vi "SRV_Build Calculated Sensors Commands.vi"(8 "error in (no error)":errorcluster, 10 "Calculated Sensors Config":T2[](array[typedef]) {"Register" format="%.0x"; "I2C Address" format="%.0x"; "Sample Period (ms)" min=10 max=60000 step=1; "Digital Mask" format="%.0x"; "Channel" format="%.0x"}, 11 "Sensor Config":T2={"Name"="", "A/D"=enum."Digital", "I2C Address"=0, "Register"=0, "Channel"=0, "Digital Mask"=0, "Units"="", "Sampling Mode"=enum."Polled", "Sample Period (ms)"=1000, "Formula"="", "Sensor View Config"={"Sensor Name"=enum."Gauge 01", "Minimum"=0.0, "Maximum"=10.0}, "Active"=FALSE, "PicoC Shared Var Type"=enum."Integer", "Index"=0, "Stream Multiple?"=FALSE, "Index End"=255, "Bytes"=enum."1 Byte", "Source Sensor Name"="", "Repeat Start"=FALSE, "Integer Word Type"=enum."Unsigned", "Byte Swap"=FALSE} {"Register" format="%.0x"; "I2C Address" format="%.0x"; "Sample Period (ms)" min=10 max=60000 step=1; "Digital Mask" format="%.0x"; "Channel" format="%.0x"}) -> (0 "error out":errorcluster, 1 "Calculated Sensors Array":T1[](array[typedef]) {"Parsed Formula"."Y Values" format="%.2f"; "Sensor Config"."Register" format="%.0x"; "Sensor Config"."I2C Address" format="%.0x"; "Sensor Config"."Sample Period (ms)" min=10 max=60000 step=1; "Sensor Config"."Digital Mask" format="%.0x"; "Sensor Config"."Channel" format="%.0x"}, 3 "Sensor Config dup":T2={"Name"="", "A/D"=enum."Digital", "I2C Address"=0, "Register"=0, "Channel"=0, "Digital Mask"=0, "Units"="", "Sampling Mode"=enum."Polled", "Sample Period (ms)"=1000, "Formula"="", "Sensor View Config"={"Sensor Name"=enum."Gauge 01", "Minimum"=0.0, "Maximum"=10.0}, "Active"=FALSE, "PicoC Shared Var Type"=enum."Integer", "Index"=0, "Stream Multiple?"=FALSE, "Index End"=255, "Bytes"=enum."1 Byte", "Source Sensor Name"="", "Repeat Start"=FALSE, "Integer Word Type"=enum."Unsigned", "Byte Swap"=FALSE} {"Register" format="%.0x"; "I2C Address" format="%.0x"; "Sample Period (ms)" min=10 max=60000 step=1; "Digital Mask" format="%.0x"; "Channel" format="%.0x"})   [LabVIEW 2009]
uses:
  SRV_Sensor Config Cluster.ctl
  SRV_Sensor Analog-Digital.ctl
  SRV_Sensor Sampling Mode.ctl
  SRV_Sensor View Config Cluster.ctl
  SRV_Sensors Names.ctl
  SRV_Sensor PicoC Shared Var Type.ctl
  SRV_Sensor Number of Bytes.ctl
  SRV_Sensor Integer Word Type.ctl
  SRV_Calculated Sensor Cfg.ctl
panel:
  # "operator"
  # "register1"
  # "register2"
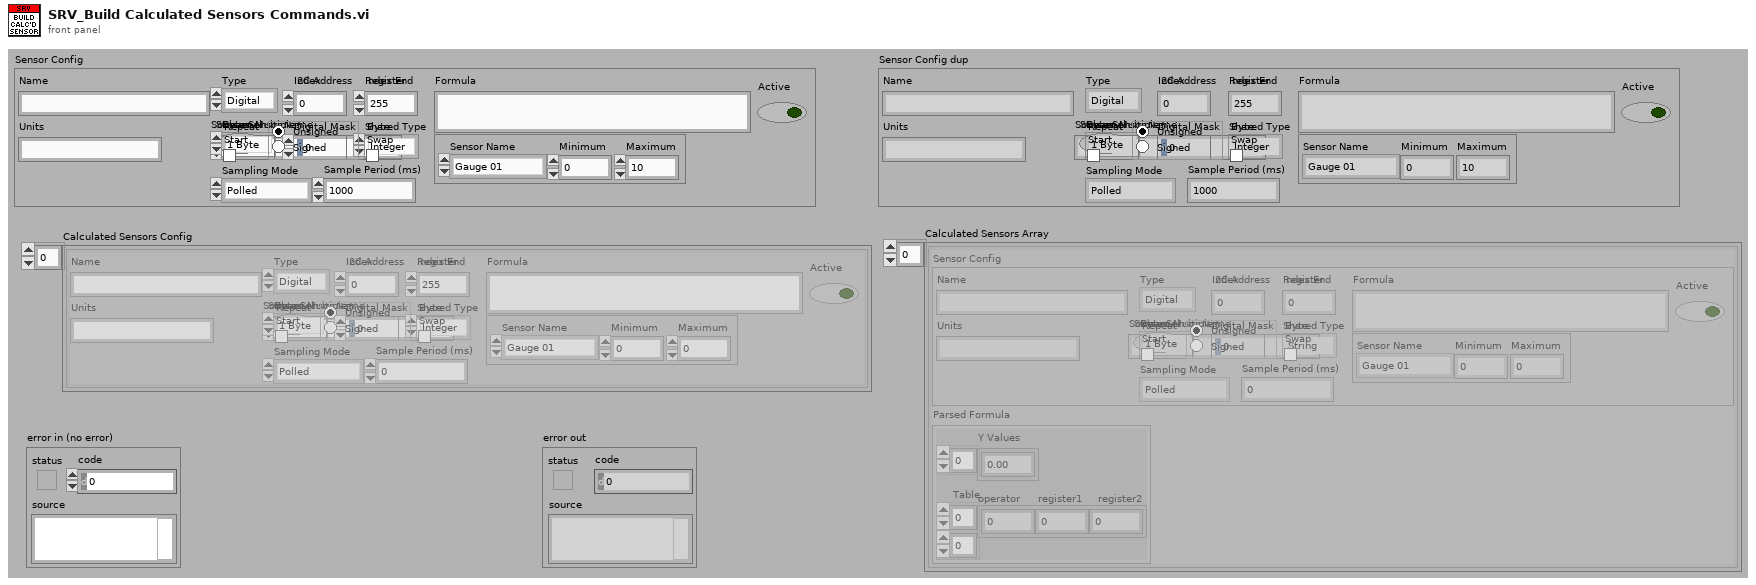
[diagram p1: front panel]
types:
  T1 = typedef "SRV_Calculated Sensor Cfg.ctl" = cluster{"Sensor Config":T2, "Parsed Formula":cluster{"Table":i32[][], "Y Values":dbl[]}}
  T2 = typedef "SRV_Sensor Config Cluster.ctl" = cluster{"Name":string, "A/D":T3, "I2C Address":u8, "Register":u8, "Channel":u8, "Digital Mask":u16, "Units":string, "Sampling Mode":T4, "Sample Period (ms)":u32, "Formula":string, "Sensor View Config":T5, "Active":bool, "PicoC Shared Var Type":T7, "Index":u8, "Stream Multiple?":bool, "Index End":u8, "Bytes":T8, "Source Sensor Name":string, "Repeat Start":bool, "Integer Word Type":T9, "Byte Swap":bool}
  T3 = typedef "SRV_Sensor Analog-Digital.ctl" = enum16{"Digital", "Analog", "PicoC Shared", "Calculated"}
  T4 = typedef "SRV_Sensor Sampling Mode.ctl" = enum16{"Polled", "Streaming"}
  T5 = typedef "SRV_Sensor View Config Cluster.ctl" = cluster{"Sensor Name":T6, "Minimum":dbl, "Maximum":dbl}
  T6 = typedef "SRV_Sensors Names.ctl" = enum16{"Gauge 01", "Gauge 02", "Gauge 03", "Gauge 04", "Meter 01", "Meter 02", "Meter 03", "Meter 04", "Numeric 01", "Numeric 02", "Numeric 03", "Numeric 04", "Numeric 05", "Numeric 06", "Numeric 07", "Numeric 08", "Boolean 01", "Boolean 02", "Boolean 03", "Boolean 04", "Boolean 05", "Boolean 06", "Boolean 07", "Boolean 08", "Boolean 09", "Boolean 10", "Boolean 11", "Boolean 12", "Boolean 13", "Boolean 14", "Boolean 15", "Boolean 16", "Boolean 17", "Boolean 18", "Boolean 19", "Boolean 20", "Boolean 21", "Boolean 22", "Boolean 23", "Boolean 24", "Boolean 25", "Boolean 26", "Boolean 27", "Boolean 28", "Boolean 29", "Boolean 30", "Boolean 31", "Boolean 32"}
  T7 = typedef "SRV_Sensor PicoC Shared Var Type.ctl" = enum16{"String", "Integer", "Float"}
  T8 = typedef "SRV_Sensor Number of Bytes.ctl" = enum16{"1 Byte", "2 Bytes"}
  T9 = typedef "SRV_Sensor Integer Word Type.ctl" = enum32{"Unsigned", "Signed"}
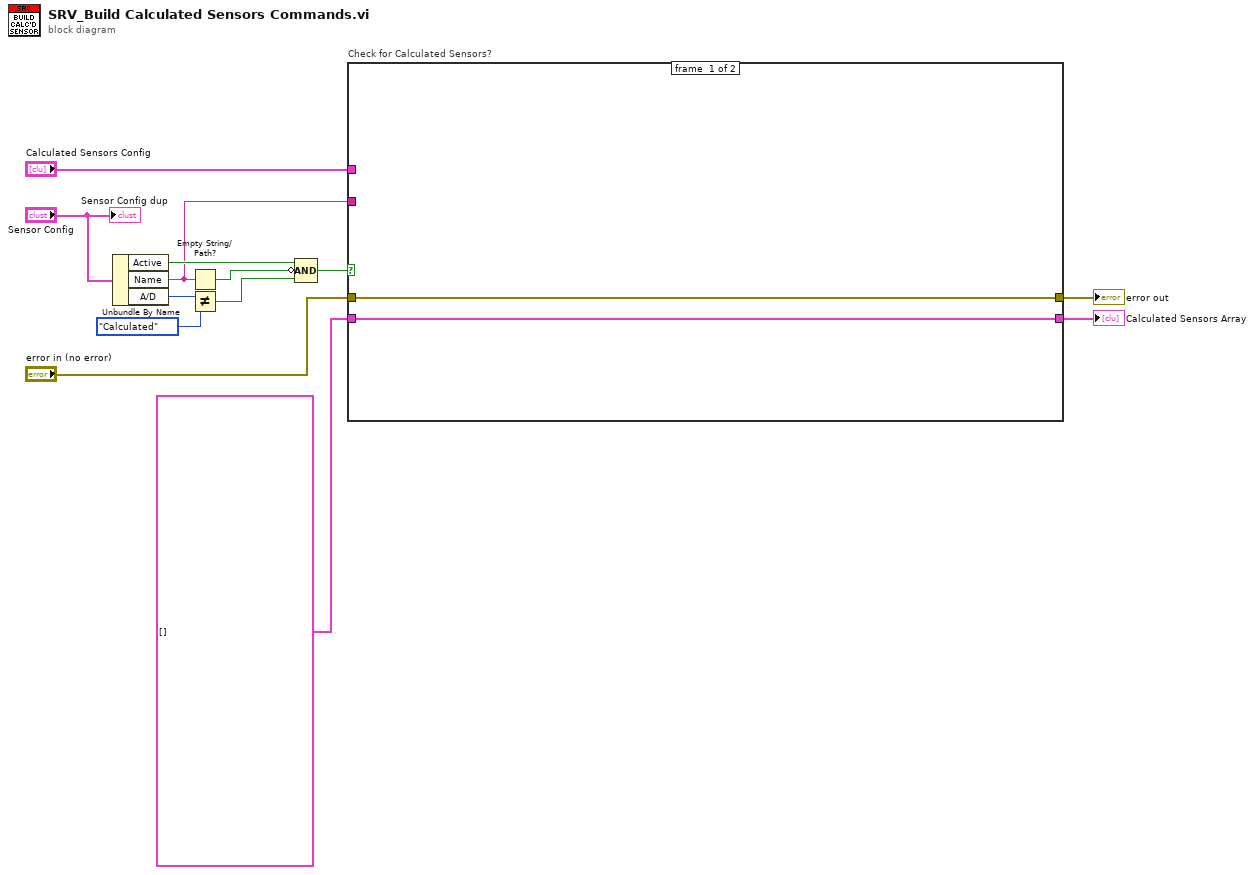
[diagram p0: block diagram]
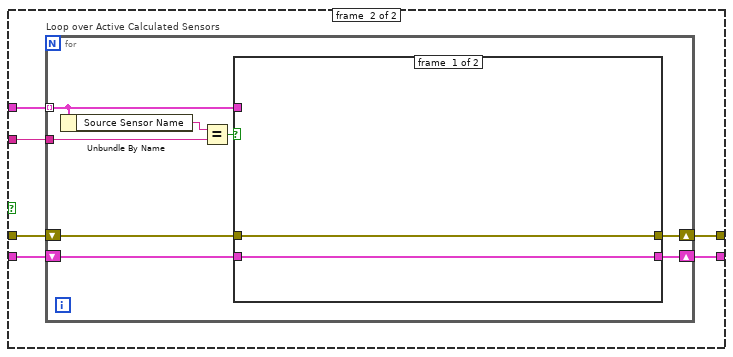
[diagram p2: hidden frame]
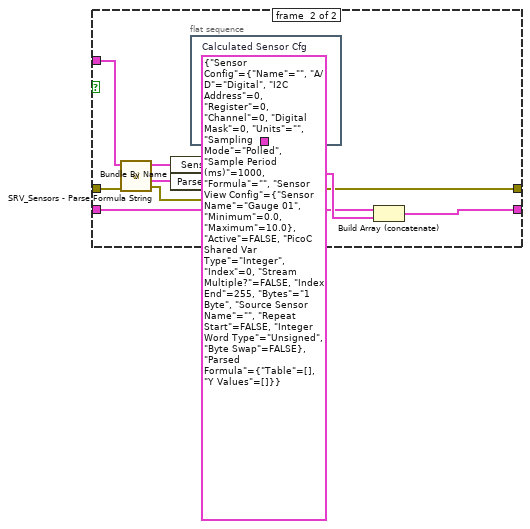
[diagram p3: hidden frame]
diagram:
  n1 = Unbundle By Name("Sensor Config") -> ("Active"=w12:bool, "Name"=w5:string, "A/D"=w10:T3)
  n2 = Empty String/Path?(string/path=w5) -> (empty?=w11:bool)
  n3 = Not Equal?(x=w10, y=SRV_Sensor_Analog-Digital."Calculated") -> (x != y?=w8:bool)
  n4 = Compound Arithmetic op=AND(w12, invert w11, w8) -> (w7:bool)
  n5 = case "Check for Calculated Sensors?" shown="True" w7 {
    tunnel: "Calculated Sensors Config" -> [_ w21]
    tunnel: w5 -> [_ w20]
    tunnel: [w15 w19] -> w4
    tunnel: T1[] [] ("Calculated Sensors Array") -> [w15 w18]
    tunnel: "error in (no error)" -> [w14 w17]
    tunnel: [w14 w16] -> w1
    frame #0 {
    }
    frame #1 {
      n6 = for "Loop over Active Calculated Sensors" {
        tunnel: w21 -> [w26] mode=indexing
        tunnel: w20 -> [w28]
        shift-right: [w24] -> w19
        shift-left: w18 -> [w25]
        shift-right: [w22] -> w16
        shift-left: w17 -> [w23]
        n7 = Unbundle By Name(w26) -> ("Source Sensor Name"=w29:string)
        n8 = Equal?(x=w29, y=w28) -> (x = y?=w27:bool)
        n9 = case shown="True" w27 {
          tunnel: w26 -> [_ w40]
          tunnel: w25 -> [w31 w35]
          tunnel: [w31 w34] -> w24
          tunnel: w23 -> [w30 w33]
          tunnel: [w30 w32] -> w22
          frame #0 {
          }
          frame #1 {
            n10 = call "SRV_Sensors - Parse Formula String.vi"("error in (no error)"=w33, "Sensor Config"=w40) -> ("error out"=w32:errorcluster, "Parsed Formula"=w37:cluster{"Table":i32[][], "Y Values":dbl[]}, "Sensor Config out"=w38:T2)  [unwired: 7 in]
            n11 = Bundle By Name(cluster=w39, "Sensor Config"=w38, "Parsed Formula"=w37) -> (w36:T1)
            n12 = flat-sequence {
              tunnel: [w41] -> w39
              frame #0 {
                w41 = T1 {"Sensor Config"={"Name"="", "A/D"=enum."Digital", "I2C Address"=0, "Register"=0, "Channel"=0, "Digital Mask"=0, "Units"="", "Sampling Mode"=enum."Polled", "Sample Period (ms)"=1000, "Formula"="", "Sensor View Config"={"Sensor Name"=enum."Gauge 01", "Minimum"=0.0, "Maximum"=10.0}, "Active"=FALSE, "PicoC Shared Var Type"=enum."Integer", "Index"=0, "Stream Multiple?"=FALSE, "Index End"=255, "Bytes"=enum."1 Byte", "Source Sensor Name"="", "Repeat Start"=FALSE, "Integer Word Type"=enum."Unsigned", "Byte Swap"=FALSE}, "Parsed Formula"={"Table"=[], "Y Values"=[]}}  # Calculated Sensor Cfg
              }
            }
            n13 = Build Array (concatenate)(w35, w36) -> (w34:T1[])
          }
        }
      }
    }
  }
  "error out" <- w1
  "Calculated Sensors Array" <- w4
  "Sensor Config dup" <- "Sensor Config"
